vi "EL-RIO-CM v1.0 Register DI IRQ.vi"(4 "Callback VI Reference":T2, 5 "Allow Overwrite Operation? (F)":bool, 6 "Edge Count":u32, 7 "IRQ Number":u8, 8 "error in (no error)":errorcluster, 9 "Digital Interrupt Type":T3, 10 "Channel Name":string, 11 "Resource name":T1 caption="RIO Device") -> (0 "error out":errorcluster)   [LabVIEW 2021]
uses:
  <vilib>/myRIO/Common/Instrument Driver Framework/myRIO v1.0/IRQ/typedefs/DI IRQ Type.ctl
  <vilib>/myRIO/Common/Instrument Driver Framework/myRIO v1.0/IRQ/typedefs/Callback VI Ref.ctl
  <vilib>/userDefined/High Color/nirio_resource_hc.ctl
  <vilib>/myRIO/Common/Instrument Driver Framework/EL-RIO-CM v1.0/IRQ/typedefs/EL-RIO-CM v1.0 DI IRQ Channels Enum.ctl
  <vilib>/myRIO/Common/Instrument Driver Framework/myRIO v1.0/IRQ/typedefs/IRQ Type.ctl
  <vilib>/myRIO/Common/Instrument Driver Framework/myRIO v1.0/IRQ/typedefs/IO IRQ Channels Enum.ctl
  <vilib>/Utility/VariantDataType/GetNumericInfo.vi
  <vilib>/Utility/error.llb/Error Cluster From Error Code.vi
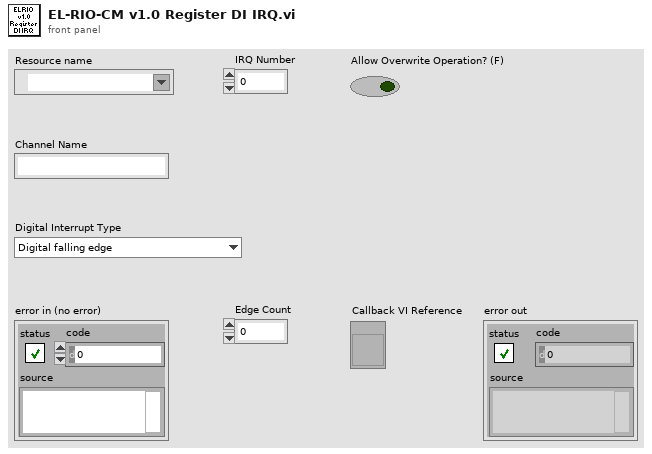
[diagram p1: front panel]
types:
  T1 = typedef "nirio_resource_hc.ctl" = tag
  T2 = typedef "Callback VI Ref.ctl" = refnum<vi>
  T3 = typedef "DI IRQ Type.ctl" = enum16{"Digital falling edge", "Digital rising edge", "Digital edge"}
  T4 = typedef "EL-RIO-CM v1.0 DI IRQ Channels Enum.ctl" = enum16{"Not Connected", "A/DIO0 (Interrupt)", "A/DIO1 (Interrupt)", "A/DIO2 (Interrupt)", "A/DIO3 (Interrupt)", "Button0 (Interrupt)"}
  T5 = typedef "IRQ Type.ctl" = enum16{"Timer", "Analog falling edge", "Analog rising edge", "Digital falling edge", "Digital rising edge", "Digital edge"}
  T6 = typedef "IO IRQ Channels Enum.ctl" = enum16{"Not Connected", "A/AI0 (Interrupt)", "A/AI1 (Interrupt)", "A/DIO0 (Interrupt)", "A/DIO1 (Interrupt)", "A/DIO2 (Interrupt)", "A/DIO3 (Interrupt)", "Button0 (Interrupt)", "B/AI0 (Interrupt)", "B/AI1 (Interrupt)", "B/DIO0 (Interrupt)", "B/DIO1 (Interrupt)", "B/DIO2 (Interrupt)", "B/DIO3 (Interrupt)"}
  T7 = typedef "Generic FPGA Reference.ctl" = refnum<k20>
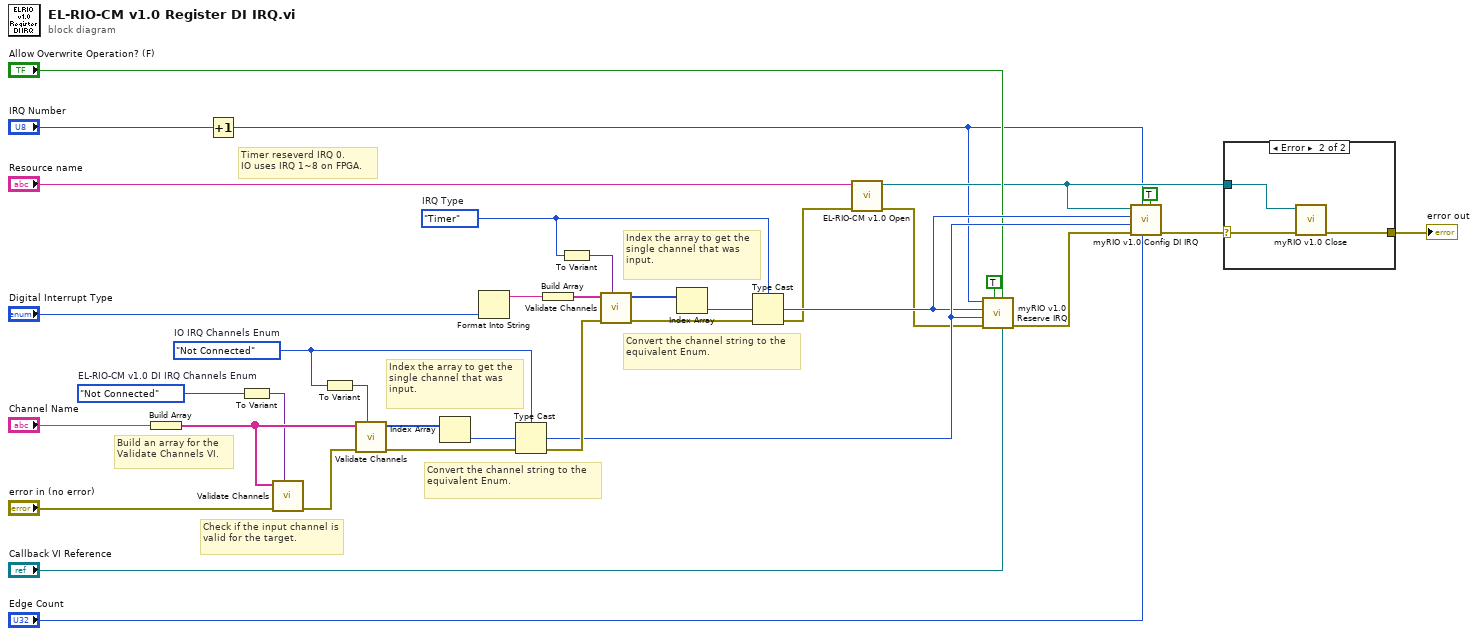
[diagram p0: block diagram]
diagram:
  w11 = EL-RIO-CM_v1.0_DI_IRQ_Channels_Enum."Not Connected"  # EL-RIO-CM v1.0 DI IRQ Channels Enum
  w22 = IRQ_Type."Timer"  # IRQ Type
  w26 = IO_IRQ_Channels_Enum."Not Connected"  # IO IRQ Channels Enum
  # "Timer reseverd IRQ 0.\nIO uses IRQ 1~8 on FPGA."
  # "Index the array to get the single channel that was input."
  # "Convert the channel string to the equivalent Enum."
  # "Index the array to get the single channel that was input."
  # "Build an array for the Validate Channels VI."
  # "Convert the channel string to the equivalent Enum."
  # "Check if the input channel is valid for the target."
  n1 = Build Array("Channel Name") -> (w32:string[])
  n2 = Increment(x="IRQ Number") -> (x+1=w2:u8)
  n3 = To Variant(anything=w11) -> (Variant=w28:variant)
  n4 = call <vilib>:"Validate Channels.vi"("Channels Enum Variant"=w28, "error in (no error)"="error in (no error)", "Channel Names"=w32) -> ("error out"=w31:errorcluster)  [unwired: 7 in, 1 out]
  n5 = To Variant(anything=w26) -> (Variant=w27:variant)
  n6 = call <vilib>:"Validate Channels.vi"("Channels Enum Variant"=w27, "error in (no error)"=w31, "Channel Names"=w32) -> ("error out"=w20:errorcluster, "Index Array"=w33:u16[])  [unwired: 7 in]
  n7 = Index Array(array=w33) -> (element=w34:u16)  [unwired: 1 in]
  n8 = Format Into String("Digital Interrupt Type") -> (resulting string=w3:string)  [unwired: 3 in, 1 out]
  n9 = Type Cast(type=w26, x=w34) -> (*(type *) &x=w17:T6)
  n10 = Build Array(w3) -> (w21:string[])
  n11 = To Variant(anything=w22) -> (Variant=w25:variant)
  n12 = call <vilib>:"Validate Channels.vi"("Channels Enum Variant"=w25, "error in (no error)"=w20, "Channel Names"=w21) -> ("error out"=w8:errorcluster, "Index Array"=w24:u16[])  [unwired: 7 in]
  n13 = Index Array(array=w24) -> (element=w23:u16)  [unwired: 1 in]
  n14 = Type Cast(type=w22, x=w23) -> (*(type *) &x=w16:T5)
  n15 = call <vilib>:"EL-RIO-CM v1.0 Open.vi"("error in (no error)"=w8, "Resource name"="Resource name") -> ("error out"=w7:errorcluster, "myRIO FPGA Ref Out"=w6:T7)  [unwired: 8 in]
  n16 = call <vilib>:"myRIO v1.0 Reserve IRQ.vi"("Callback VI Ref"="Callback VI Reference", "Allow Overwrite? (F)"="Allow Overwrite Operation? (F)", "Is Reserve?"=TRUE, "error in (no error)"=w7, "IO IRQ Channels Enum"=w17, "IRQ Type"=w16, "IRQ Number"=w2) -> ("error out"=w18:errorcluster)  [unwired: 3 in, 1 out]
  n17 = call <vilib>:"myRIO v1.0 Config DI IRQ.vi"("Enable IRQ?"=TRUE, "Edge Count"="Edge Count", "IRQ Number"=w2, "error in (no error)"=w18, "IO IRQ Channels Enum"=w17, "IRQ Type"=w16, "myRIO FPGA Ref In"=w6) -> ("error out"=w13:errorcluster)  [unwired: 4 in]
  n18 = case shown="Error" w13 {
    selector: w13 -> [w35 w38]
    tunnel: w6 -> [_ w36]
    tunnel: [w35 w37] -> w12
    frame No Error {
    }
    frame Error {
      n19 = call <vilib>:"myRIO v1.0 Close.vi"("error in (no error)"=w38, "myRIO FPGA Ref In"=w36) -> ("error out"=w37:errorcluster)  [unwired: 9 in]
    }
  }
  "error out" <- w12
